vi "Keithley 2260B Examples.vi"() -> ()   [LabVIEW 2009]
doc: "This example shows how to configure the instrument's output voltage level, over current protection, and over voltage protection. The actual voltage level and actual current level are returned as well as whether over voltage protection (OVP) or over current protection (OCP) has been tripped."
uses:
  <instrlib>/Keithley 2260B/Keithley 2260B.lvlib
panel:
  in  "Protection Clear":bool
  in  "Output Mode ( 0 : CVHS )":enum16{"CVHS", "CCHS", "CVLS", "CCLS"}(ring) caption="Output Mode"
  in  "I-SR Falling (1 A)":dbl=1.0 format="%.2g"
  in  "I-SR Rising (1 A)":dbl=1.0 format="%.2g"
  in  "V-SR Falling (1 V)":dbl=1.0 format="%.2g"
  in  "V-SR Rising (1 V)":dbl=1.0 format="%.2g"
  out "Protection Tripped":bool
  out "AC Power Off":bool
  out "Shutdown Tripped":bool
  out "OTP Tripped":bool
  out "OCP Tripped":bool
  out "OVP Tripped":bool
  out "Output OFF Delay":bool
  out "Output ON Delay":bool
  in  "Output OFF Delay (0.00 s)":dbl format="%.2g"
  in  "Output ON Delay (0.00 s)":dbl format="%.2g"
  in  "Output (T: Enable)":bool
  out "CC":bool
  out "CV":bool
  in  "OCP (5A)":dbl=5.0 format="%.3g"
  in  "Serial Configuration":T1={"Baud Rate"=9600, "Parity"=0, "Data Bits"=8, "Stop Bits"=10, "Flow Control"=0} {"Flow Control" items=["None", "XON/XOFF", "RTS/CTS", "XON/XOFF & RTS/CTS", "DTR/DSR", "XON/XOFF & DTR/DSR"]; "Stop Bits" items=["1.0"=10, "1.5"=15, "2.0"=20]; "Data Bits" items=["7"=7, "8"=8]; "Parity" items=["None", "Odd", "Even", "Mark", "Space"]; "Baud Rate" items=["300"=300, "600"=600, "1200"=1200, "2400"=2400, "4800"=4800, "9600"=9600, "19200"=19200]}
  in  "Stop":bool
  in  "OVP (10V)":dbl=10.0 format="%.3f"
  out "Actual Current (A)":dbl format="%.3f"
  out "Actual Voltage (V)":dbl format="%.3f"
  in  "Voltage Level (0V)":dbl format="%.3f"
  in  "Current Level (0A)":dbl format="%.3f"
  in  "VISA resource name":refnum<visa-resource-name>
  # "Voltage"
  # "Current"
  # "WARNINGS: \nThe OVP, OCP Setting range depends on the 2260A Models\nFor 80V, the minimal value is 8V(10%). The max value is 88V(110%)\nFor 30V, the minimal value is 3V(10%). The max value is 33V(110%)\nFor 36A, the minimal value is 3.60A(10%). The max value is 39.6A(110%)"
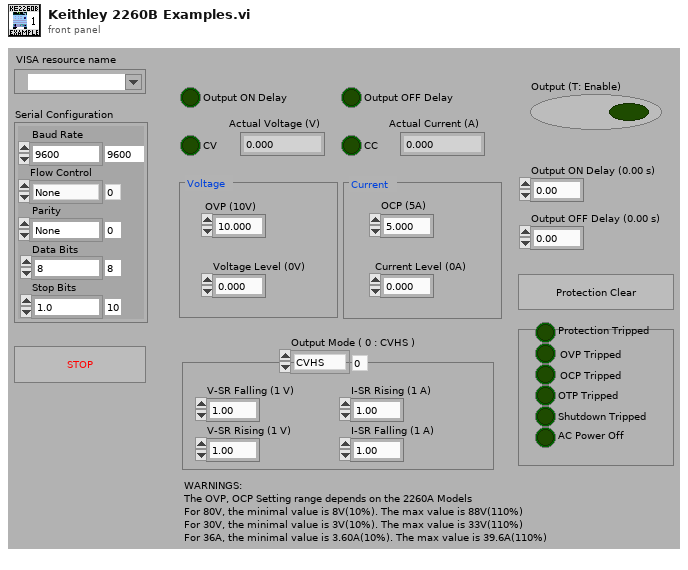
[diagram p1: front panel]
types:
  T1 = cluster{"Baud Rate":u32, "Parity":u16, "Data Bits":u16, "Stop Bits":u16, "Flow Control":u16}
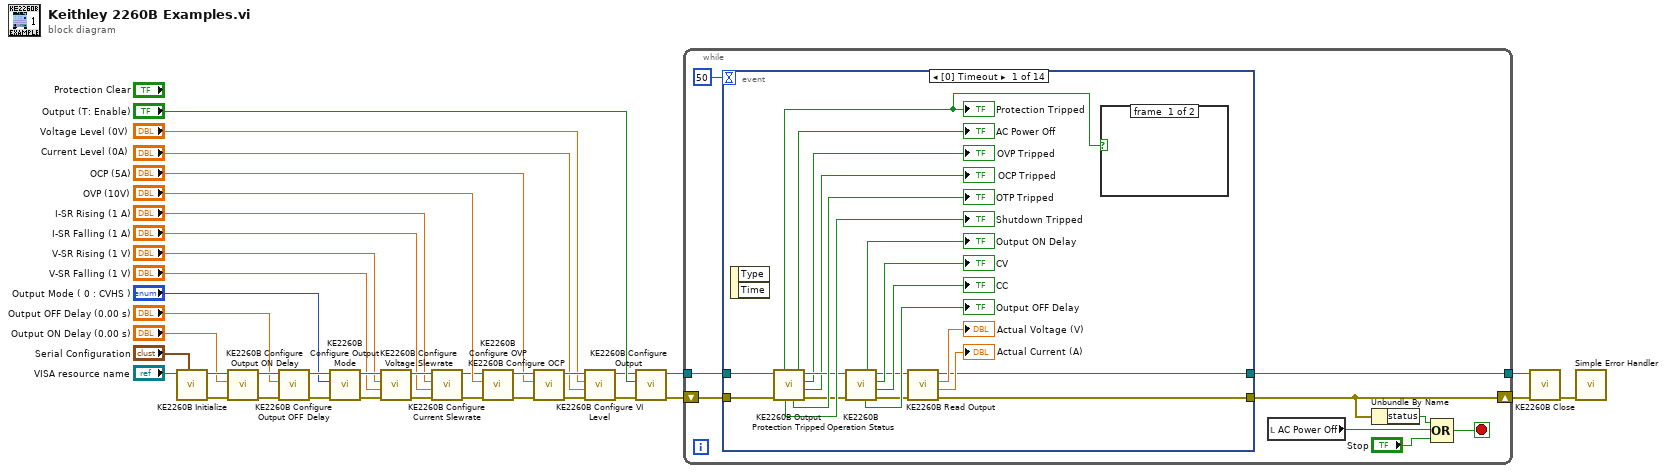
[diagram p0: block diagram]
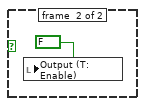
[diagram p2: hidden frame]
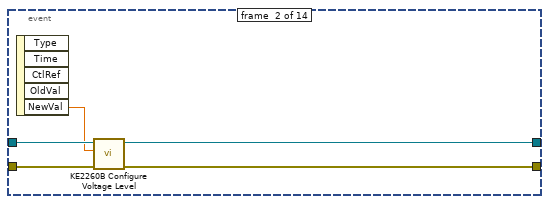
[diagram p3: hidden frame]
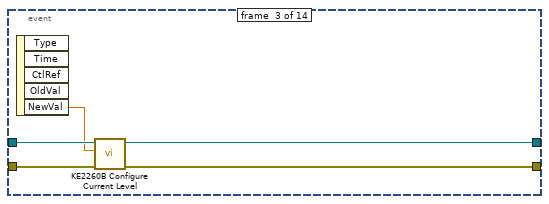
[diagram p4: hidden frame]
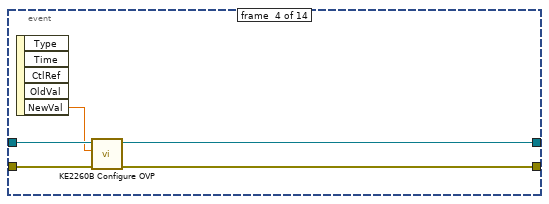
[diagram p5: hidden frame]
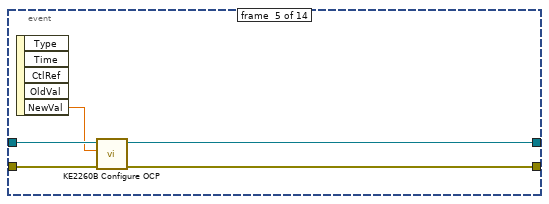
[diagram p6: hidden frame]
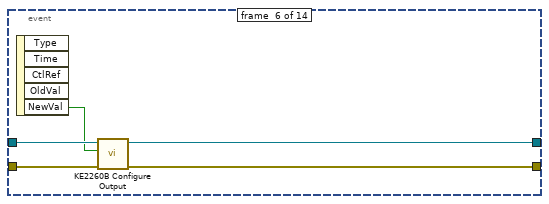
[diagram p7: hidden frame]
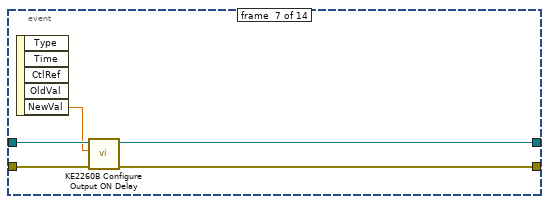
[diagram p8: hidden frame]
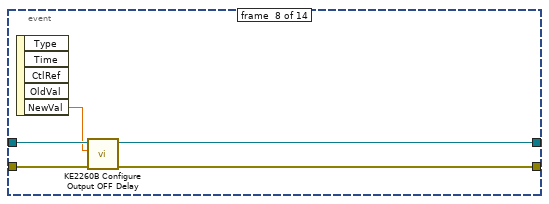
[diagram p9: hidden frame]
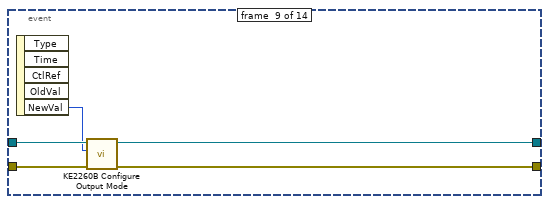
[diagram p10: hidden frame]
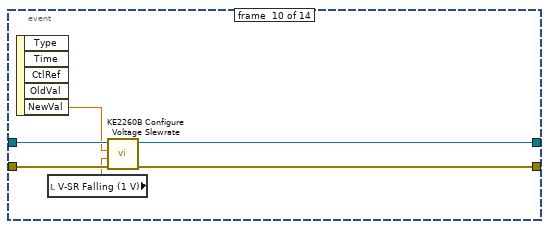
[diagram p11: hidden frame]
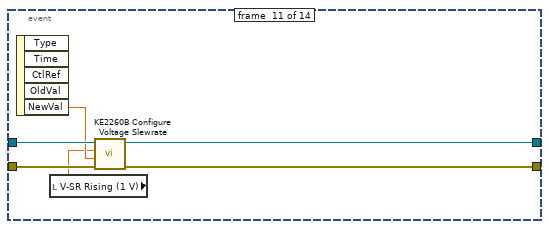
[diagram p12: hidden frame]
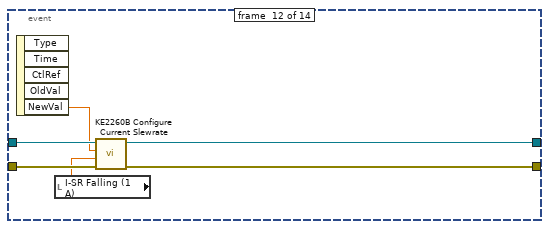
[diagram p13: hidden frame]
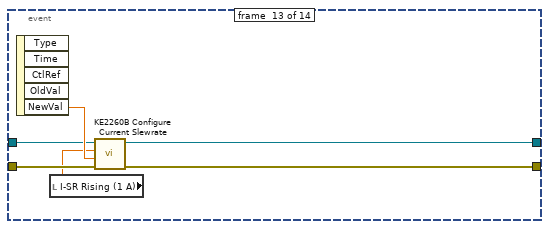
[diagram p14: hidden frame]
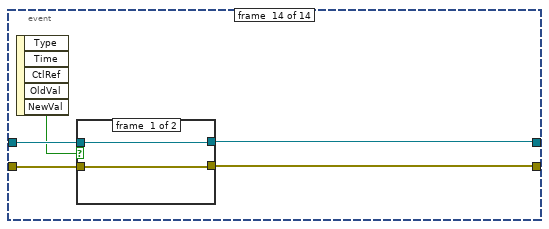
[diagram p15: hidden frame]
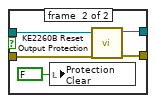
[diagram p16: hidden frame]
diagram:
  n1 = call <instrlib>:"KE2260B Initialize.vi"("Serial Configuration"="Serial Configuration", "VISA resource name"="VISA resource name") -> ("error out"=w13:errorcluster, "VISA resource name out"=w19:refnum<visa-resource-name>)  [unwired: 8 in]
  n2 = call <instrlib>:"KE2260B Configure Output ON Delay.vi"("error in (no error)"=w13, "Output ON Delay (0.00 s)"="Output ON Delay (0.00 s)", "VISA resource name"=w19) -> ("error out"=w12:errorcluster, "VISA resource name out"=w18:refnum<visa-resource-name>)  [unwired: 7 in]
  n3 = call <instrlib>:"KE2260B Configure Output OFF Delay.vi"("error in (no error)"=w12, "Output OFF Delay (0.00 s)"="Output OFF Delay (0.00 s)", "VISA resource name"=w18) -> ("error out"=w11:errorcluster, "VISA resource name out"=w17:refnum<visa-resource-name>)  [unwired: 7 in]
  n4 = call <instrlib>:"KE2260B Configure Output Mode.vi"("error in (no error)"=w11, "Output Mode ( 0 : CVHS )"="Output Mode ( 0 : CVHS )", "VISA resource name"=w17) -> ("error out"=w10:errorcluster, "VISA resource name out"=w16:refnum<visa-resource-name>)  [unwired: 7 in]
  n5 = call <instrlib>:"KE2260B Configure Voltage Slewrate.vi"("error in (no error)"=w10, "Slewrate Falling (0.01 V)"="V-SR Falling (1 V)", "Slewrate Rising (0.01 V)"="V-SR Rising (1 V)", "VISA resource name"=w16) -> ("error out"=w9:errorcluster, "VISA resource name out"=w15:refnum<visa-resource-name>)  [unwired: 6 in]
  n6 = call <instrlib>:"KE2260B Configure Current Slewrate.vi"("error in (no error)"=w9, "Slewrate Falling (0.01 A)"="I-SR Falling (1 A)", "Slewrate Rising (0.01 A)"="I-SR Rising (1 A)", "VISA resource name"=w15) -> ("error out"=w8:errorcluster, "VISA resource name out"=w14:refnum<visa-resource-name>)  [unwired: 6 in]
  n7 = call <instrlib>:"KE2260B Configure OVP.vi"("error in (no error)"=w8, "OVP (0.000 V)"="OVP (10V)", "VISA resource name"=w14) -> ("error out"=w31:errorcluster, "VISA resource name out"=w30:refnum<visa-resource-name>)  [unwired: 7 in]
  n8 = call <instrlib>:"KE2260B Configure OCP.vi"("error in (no error)"=w31, "OCP (0.000 V)"="OCP (5A)", "VISA resource name"=w30) -> ("error out"=w22:errorcluster, "VISA resource name out"=w25:refnum<visa-resource-name>)  [unwired: 7 in]
  n9 = call <instrlib>:"KE2260B Configure VI Level.vi"("error in (no error)"=w22, "Current Level (0.000 A)"="Current Level (0A)", "Voltage Level (0.000 V)"="Voltage Level (0V)", "VISA resource name"=w25) -> ("error out"=w20:errorcluster, "VISA resource name out"=w21:refnum<visa-resource-name>)  [unwired: 6 in]
  n10 = call <instrlib>:"KE2260B Configure Output.vi"("error in (no error)"=w20, "Enable Output (T: Enable)"="Output (T: Enable)", "VISA resource name"=w21) -> ("error out"=w35:errorcluster, "VISA resource name out"=w36:refnum<visa-resource-name>)  [unwired: 7 in]
  n11 = while {
    tunnel: w36 -> [w46]
    tunnel: [w41] -> w27
    shift-right: [w40] -> w26
    shift-left: w35 -> [w45]
    stop <- w42 stop-if-true
    n12 = event shown="[0] Timeout" {
      selector: _ -> [_ _ _ _ _ _ _ _ _ _ _ _ _ _]
      dyn-events: _ -> [_ _ _ _ _ _ _ _ _ _ _ _ _ _]
      timeout: 50 -> [_ _ _ _ _ _ _ _ _ _ _ _ _ _]
      tunnel: [w49 w72 w75 w80 w87 w90 w96 w100 w104 w112 w118 w123 w128 w135] -> w41
      tunnel: w46 -> [w51 w70 w77 w82 w85 w92 w97 w102 w107 w113 w119 w125 w130 w136]
      tunnel: [w48 w71 w74 w79 w86 w89 w94 w99 w103 w110 w116 w122 w127 w133] -> w40
      tunnel: w45 -> [w50 w69 w76 w81 w84 w91 w95 w101 w106 w111 w117 w124 w129 w134]
      event #0 {
        n13 = event-data() -> ()  [unwired: 1 in, 2 out]
        n14 = call <instrlib>:"KE2260B Output Protection Tripped.vi"("error in (no error)"=w50, "VISA resource name"=w51) -> ("error out"=w61:errorcluster, "OCP Tripped?"=→"OCP Tripped":bool, "OVP Tripped?"=→"OVP Tripped":bool, "VISA resource name out"=w60:refnum<visa-resource-name>, "OTP Tripped?"=→"OTP Tripped":bool, "AC Power Off?"=→"AC Power Off":bool, "Shutdown Tripped?"=→"Shutdown Tripped":bool, "Protection Tripped?"=w47:bool)  [unwired: 2 in]
        "Protection Tripped" <- w47
        n15 = call <instrlib>:"KE2260B Operation Status.vi"("error in (no error)"=w61, "VISA resource name"=w60) -> ("error out"=w55:errorcluster, "CC"=→"CC":bool, "CV"=→"CV":bool, "VISA resource name out"=w54:refnum<visa-resource-name>, "Output OFF Delay"=→"Output OFF Delay":bool, "Output ON Delay"=→"Output ON Delay":bool)  [unwired: 4 in]
        n16 = call <instrlib>:"KE2260B Read Output.vi"("error in (no error)"=w55, "VISA resource name"=w54) -> ("error out"=w48:errorcluster, "Actual Current Level (A)"=→"Actual Current (A)":dbl, "Actual Voltage Level (V)"=→"Actual Voltage (V)":dbl, "VISA resource name out"=w49:refnum<visa-resource-name>)  [unwired: 6 in]
        n17 = case shown="True" w47 {
          frame #0 {
          }
          frame #1 {
            n18 = local write "Output (T: Enable)"(FALSE) -> ()
          }
        }
      }
      event #1 {
        n19 = event-data() -> ("NewVal"=w68:dbl)  [unwired: 1 in, 4 out]
        n20 = call <instrlib>:"KE2260B Configure Voltage Level.vi"("error in (no error)"=w69, "Voltage Level (0.000 V)"=w68, "VISA resource name"=w70) -> ("error out"=w71:errorcluster, "VISA resource name out"=w72:refnum<visa-resource-name>)  [unwired: 7 in]
      }
      event #2 {
        n21 = event-data() -> ("NewVal"=w73:dbl)  [unwired: 1 in, 4 out]
        n22 = call <instrlib>:"KE2260B Configure Current Level.vi"("error in (no error)"=w76, "Current Level (0.000 A)"=w73, "VISA resource name"=w77) -> ("error out"=w74:errorcluster, "VISA resource name out"=w75:refnum<visa-resource-name>)  [unwired: 7 in]
      }
      event #3 {
        n23 = event-data() -> ("NewVal"=w78:dbl)  [unwired: 1 in, 4 out]
        n24 = call <instrlib>:"KE2260B Configure OVP.vi"("error in (no error)"=w81, "OVP (0.000 V)"=w78, "VISA resource name"=w82) -> ("error out"=w79:errorcluster, "VISA resource name out"=w80:refnum<visa-resource-name>)  [unwired: 7 in]
      }
      event #4 {
        n25 = event-data() -> ("NewVal"=w83:dbl)  [unwired: 1 in, 4 out]
        n26 = call <instrlib>:"KE2260B Configure OCP.vi"("error in (no error)"=w84, "OCP (0.000 V)"=w83, "VISA resource name"=w85) -> ("error out"=w86:errorcluster, "VISA resource name out"=w87:refnum<visa-resource-name>)  [unwired: 7 in]
      }
      event #5 {
        n27 = event-data() -> ("NewVal"=w88:bool)  [unwired: 1 in, 4 out]
        n28 = call <instrlib>:"KE2260B Configure Output.vi"("error in (no error)"=w91, "Enable Output (T: Enable)"=w88, "VISA resource name"=w92) -> ("error out"=w89:errorcluster, "VISA resource name out"=w90:refnum<visa-resource-name>)  [unwired: 7 in]
      }
      event #6 {
        n29 = event-data() -> ("NewVal"=w93:dbl)  [unwired: 1 in, 4 out]
        n30 = call <instrlib>:"KE2260B Configure Output ON Delay.vi"("error in (no error)"=w95, "Output ON Delay (0.00 s)"=w93, "VISA resource name"=w97) -> ("error out"=w94:errorcluster, "VISA resource name out"=w96:refnum<visa-resource-name>)  [unwired: 7 in]
      }
      event #7 {
        n31 = event-data() -> ("NewVal"=w98:dbl)  [unwired: 1 in, 4 out]
        n32 = call <instrlib>:"KE2260B Configure Output OFF Delay.vi"("error in (no error)"=w101, "Output OFF Delay (0.00 s)"=w98, "VISA resource name"=w102) -> ("error out"=w99:errorcluster, "VISA resource name out"=w100:refnum<visa-resource-name>)  [unwired: 7 in]
      }
      event #8 {
        n33 = event-data() -> ("NewVal"=w105:enum16{"CVHS", "CCHS", "CVLS", "CCLS"})  [unwired: 1 in, 4 out]
        n34 = call <instrlib>:"KE2260B Configure Output Mode.vi"("error in (no error)"=w106, "Output Mode ( 0 : CVHS )"=w105, "VISA resource name"=w107) -> ("error out"=w103:errorcluster, "VISA resource name out"=w104:refnum<visa-resource-name>)  [unwired: 7 in]
      }
      event #9 {
        n35 = event-data() -> ("NewVal"=w109:dbl)  [unwired: 1 in, 4 out]
        n36 = local read "V-SR Falling (1 V)"() -> (w108:dbl)
        n37 = call <instrlib>:"KE2260B Configure Voltage Slewrate.vi"("error in (no error)"=w111, "Slewrate Falling (0.01 V)"=w108, "Slewrate Rising (0.01 V)"=w109, "VISA resource name"=w113) -> ("error out"=w110:errorcluster, "VISA resource name out"=w112:refnum<visa-resource-name>)  [unwired: 6 in]
      }
      event #10 {
        n38 = event-data() -> ("NewVal"=w115:dbl)  [unwired: 1 in, 4 out]
        n39 = local read "V-SR Rising (1 V)"() -> (w114:dbl)
        n40 = call <instrlib>:"KE2260B Configure Voltage Slewrate.vi"("error in (no error)"=w117, "Slewrate Falling (0.01 V)"=w115, "Slewrate Rising (0.01 V)"=w114, "VISA resource name"=w119) -> ("error out"=w116:errorcluster, "VISA resource name out"=w118:refnum<visa-resource-name>)  [unwired: 6 in]
      }
      event #11 {
        n41 = event-data() -> ("NewVal"=w121:dbl)  [unwired: 1 in, 4 out]
        n42 = local read "I-SR Falling (1 A)"() -> (w120:dbl)
        n43 = call <instrlib>:"KE2260B Configure Current Slewrate.vi"("error in (no error)"=w124, "Slewrate Falling (0.01 A)"=w120, "Slewrate Rising (0.01 A)"=w121, "VISA resource name"=w125) -> ("error out"=w122:errorcluster, "VISA resource name out"=w123:refnum<visa-resource-name>)  [unwired: 6 in]
      }
      event #12 {
        n44 = event-data() -> ("NewVal"=w131:dbl)  [unwired: 1 in, 4 out]
        n45 = local read "I-SR Rising (1 A)"() -> (w126:dbl)
        n46 = call <instrlib>:"KE2260B Configure Current Slewrate.vi"("error in (no error)"=w129, "Slewrate Falling (0.01 A)"=w131, "Slewrate Rising (0.01 A)"=w126, "VISA resource name"=w130) -> ("error out"=w127:errorcluster, "VISA resource name out"=w128:refnum<visa-resource-name>)  [unwired: 6 in]
      }
      event #13 {
        n47 = event-data() -> ("NewVal"=w132:bool)  [unwired: 1 in, 4 out]
        n48 = case shown="True" w132 {
          tunnel: w136 -> [w138 w143]
          tunnel: [w138 w142] -> w135
          tunnel: w134 -> [w137 w141]
          tunnel: [w137 w140] -> w133
          frame #0 {
          }
          frame #1 {
            n49 = local write "Protection Clear"(FALSE) -> ()
            n50 = call <instrlib>:"KE2260B Reset Output Protection.vi"("error in (no error)"=w141, "VISA resource name"=w143) -> ("error out"=w140:errorcluster, "VISA resource name out"=w142:refnum<visa-resource-name>)  [unwired: 8 in]
          }
        }
      }
    }
    n51 = local read "AC Power Off"() -> (w38:bool)
    n52 = Unbundle By Name(w40) -> ("status"=w39:bool)
    n53 = Compound Arithmetic op=OR(w39, w38, "Stop") -> (w42:bool)
  }
  n54 = call <instrlib>:"KE2260B Close.vi"("error in (no error)"=w26, "VISA resource name"=w27) -> ("error out"=w34:errorcluster)  [unwired: 9 in]
  n55 = call <vilib>:"Simple Error Handler.vi"("error in (no error)"=w34) -> ()  [unwired: 4 in, 5 out]
